vi "Database Tester.vi"(8 "error in (no error)":errorcluster, 10 "SQL query":string="SELECT * FROM ltt.daq_configuration;") -> (0 "error out":errorcluster, 3 "Database out":refnum<class "Database.lvclass">)   [LabVIEW 2023, in "HardwareAbstractionLayer_LVOOP.lvlib" / "Database.lvclass"]
uses:
  Database.lvclass
  Control/DB Options.ctl
  <vilib>/Utility/file.llb/Write Delimited Spreadsheet (string).vi
panel:
  out "data":string[][](array[string])
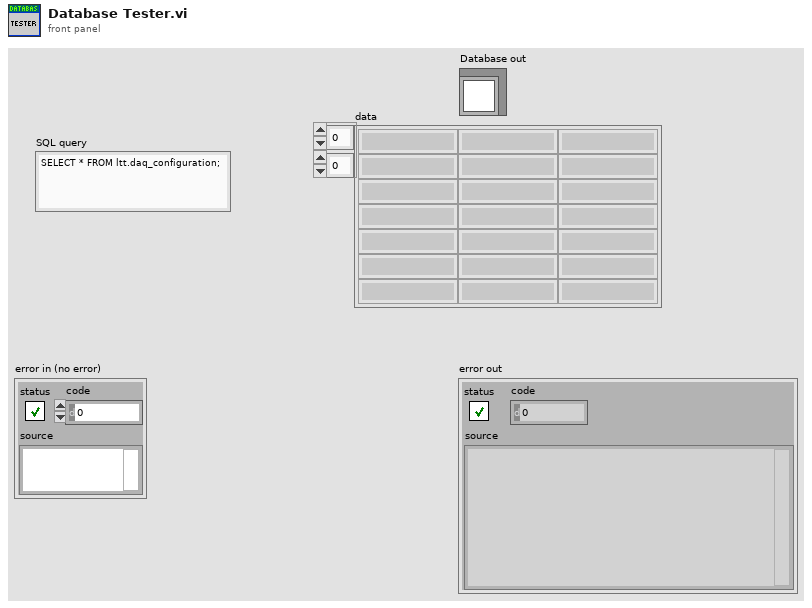
[diagram p1: front panel]
types:
  T1 = typedef "HardwareAbstractionLayer_LVOOP.lvlib/Database.lvclass/DB Options.ctl" = enum16{"Init", "Select Data", "Insert Data", "Update Data", "Delete Data", "Execute Query", "Create Schema", "Create Table", "List Tables", "List Columns", "Close"}
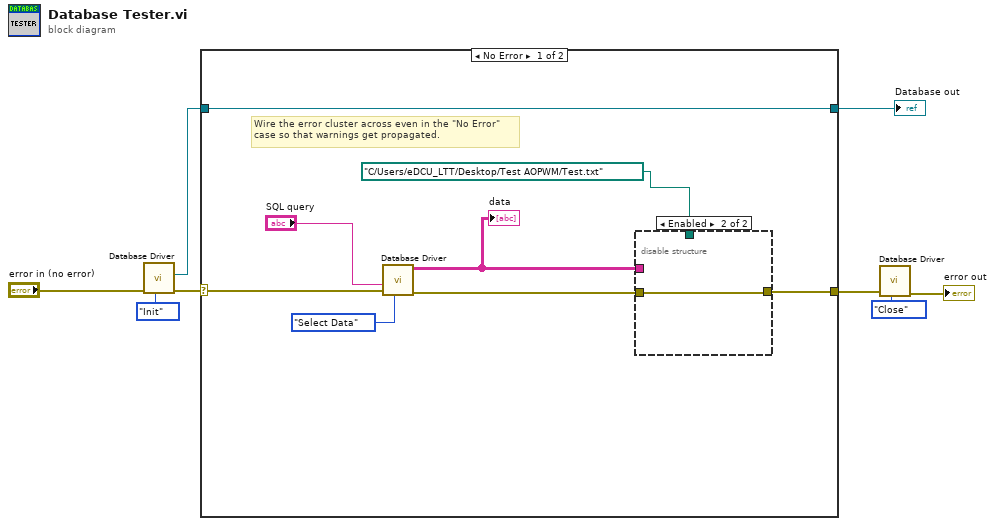
[diagram p0: block diagram]
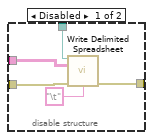
[diagram p2: hidden frame]
diagram:
  n1 = call "Database Driver.vi"("Options"=DB_Options."Init", "error in"="error in (no error)") -> ("error out"=w6:errorcluster, "Database out"=w2:refnum<class "Database.lvclass">)  [unwired: 6 in, 2 out]
  n2 = case shown="No Error" w6 {
    selector: w6 -> [w16 w24]
    tunnel: [w10 w24] -> w5
    tunnel: [w15 w23] -> w8
    tunnel: w2 -> [w15 w23]
    frame No Error {
      # "Wire the error cluster across even in the \"No Error\"\ncase so that warnings get propagated."
      n3 = call "Database Driver.vi"("Options"=DB_Options."Select Data", "error in"=w16, "SQL query"="SQL query") -> ("error out"=w11:errorcluster, "data"=w12:string[][])  [unwired: 5 in, 2 out]
      "data" <- w12
      n4 = disable-structure shown="Enabled" {
        disable-tunnel: path "C:/Users/eDCU_LTT/Desktop/Test AOPWM/Test.txt" ("file name") -> [w21 _]
        disable-tunnel: w12 -> [w20 _]
        disable-tunnel: w11 -> [w19 w22]
        disable-tunnel: [w18 w22] -> w10
        frame Disabled {
          n5 = call-poly <vilib>:"Write Delimited Spreadsheet.vi"("file path (dialog if empty)"=w21, "2D data"=w20, "error in (no error)"=w19, "delimiter (\\t)"="\t" ("delimiter (\\t)")) -> ("error out"=w18:errorcluster)  [unwired: 10 in, 1 out]
        }
        frame Enabled {
        }
      }
    }
    frame Error {
    }
  }
  "Database out" <- w8
  n6 = call "Database Driver.vi"("Options"=DB_Options."Close", "error in"=w5) -> ("error out"=→"error out":errorcluster)  [unwired: 6 in, 3 out]
